vi "Teleop.vi"(10 "Match Info":T1={"Autonomous Elapsed Seconds"=0.0, "TeleOp Elapsed Seconds"=0.0, "Disabled Elapsed Seconds"=0.0, "Visited Autonomous"=FALSE, "Visited TeleOp"=FALSE, "Visited Disabled"=FALSE, "Autonomous Settings"={"Autonomous Style"=enum."Independent", "VI Refnum"=refnum}}, 11 "Call Context":T2) -> ()   [LabVIEW 2019]
doc: "This VI is called for each TeleOp packet received from the DS where the robot is not disabled. It is often used to read from the joysticks and update I/O or to update setpoints for timed control loops. It should complete and return within 20 milliseconds or it may miss DS packets."
uses:
  <vilib>/Rock Robotics/WPI/DriverStation/WPI_DriverStationDerivedRobotMode.ctl
  <vilib>/Rock Robotics/WPI/DriverStation/WPI_DriverStationMatch Info.ctl
  <vilib>/Rock Robotics/WPI/Utilities/WPI_GetSetVariantRefNum.vi
  Robot Global Data.vi
  <vilib>/Rock Robotics/Network Tables/NT Write Variant.vi
  <vilib>/Rock Robotics/Network Tables/NT Write Number.vi
  <vilib>/Rock Robotics/Network Tables/NT Write String.vi
  <vilib>/Rock Robotics/Network Tables/NT Write Boolean.vi
  <vilib>/Rock Robotics/Network Tables/NT Write Numeric Array.vi
  <vilib>/Rock Robotics/Network Tables/NT Write Boolean Array.vi
panel:
  in  "Blue Cal":cluster{"R":dbl, "G":dbl, "B":dbl}={"R"=0.143, "G"=0.427, "B"=0.429} caption="Blue Calibration"
  in  "Green Cal":cluster{"R":dbl, "G":dbl, "B":dbl}={"R"=0.197, "G"=0.561, "B"=0.24} caption="Green Calibration"
  in  "Red Cal":cluster{"R":dbl, "G":dbl, "B":dbl}={"R"=0.561, "G"=0.323, "B"=0.114} caption="Red Calibration"
  in  "Yellow Cal":cluster{"R":dbl, "G":dbl, "B":dbl}={"R"=0.361, "G"=0.524, "B"=0.113} caption="Yellow Calibration"
  out "Matched Color Name":string
  out "Match Confidence":dbl
  out "Measured Color":cluster{"R":dbl, "G":dbl, "B":dbl}
  out "error out 2":errorcluster
  out "Proximity":u16(graph)
  out "Color":u32(colorbox)
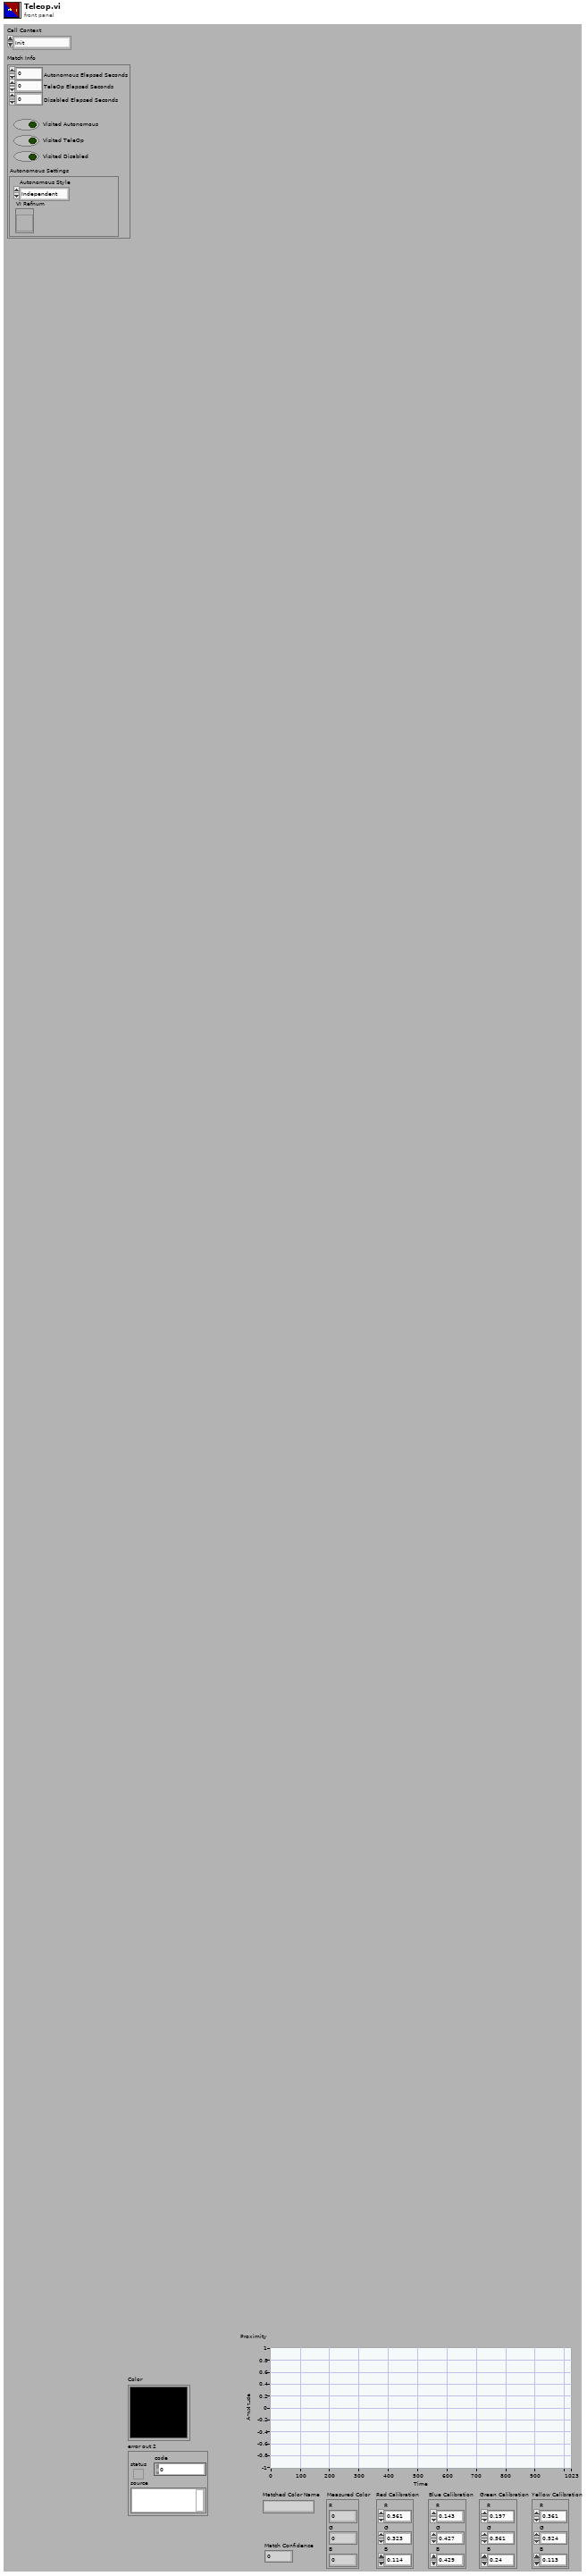
[diagram p1: front panel]
types:
  T1 = typedef "WPI_DriverStationMatch Info.ctl" = cluster{"Autonomous Elapsed Seconds":dbl, "TeleOp Elapsed Seconds":dbl, "Disabled Elapsed Seconds":dbl, "Visited Autonomous":bool, "Visited TeleOp":bool, "Visited Disabled":bool, "Autonomous Settings":cluster{"Autonomous Style":enum16{"Iterative", "Independent"}, "VI Refnum":refnum<vi>}}
  T2 = typedef "WPI_DriverStationDerivedRobotMode.ctl" = enum16{"Init", "Execute", "Stop"}
  T3 = typedef "WPI_JoystickDevRef.ctl" = cluster{"Device":T4}
  T4 = typedef "WPI_JoystickDeviceEnum.ctl" = enum16{"USB 0", "USB 1", "USB 2", "USB 3", "USB 4", "USB 5"}
  T5 = typedef "WPI_RobotDriveDevRef.ctl" = cluster{"DevStatus":errorcluster, "Motors[]":T6[], "Square Inputs":bool, "Max Output":dbl}
  T6 = typedef "WPI_MotorControlDeviceRef.ctl" = cluster{"DeviceStatus":errorcluster, "Type":T7, "PWM":cluster{"PWM Channel":T8, "DeadBand":T9}, "CAN":cluster{"Device Number":u8, "SetOutput VI Ref":variant, "GetOutput VI Ref":variant, "Enable VI Ref":variant, "Disable VI Ref":variant, "Data":variant}, "Invert":bool, "DIO PWM":cluster{"PWM \"Enable\" Channel":T8, "DIOChannel":T10, "PWM Rate":dbl}}
  T7 = typedef "WPI_MotorControlType.ctl" = enum16{"PWM", "CAN", "DIO PWM"}
  T8 = typedef "FPGA_DIOPWMChannel.ctl" = enum8{"PWM 0", "PWM 1", "PWM 2", "PWM 3", "PWM 4", "PWM 5", "PWM 6", "PWM 7", "PWM 8", "PWM 9", "PWM MXP 0", "PWM MXP 1", "PWM MXP 2", "PWM MXP 3", "PWM MXP 4", "PWM MXP 5", "PWM MXP 6", "PWM MXP 7", "PWM MXP 8", "PWM MXP 9", "Invalid"}
  T9 = typedef "WPI_PWMDeadband.ctl" = cluster{"Name":string, "maxPositivePwm":i32, "minPositivePwm":i32, "centerPwm":i32, "maxNegativePwm":i32, "minNegativePwm":i32, "angularRange":u16}
  T10 = typedef "FPGA_DIOChannel.ctl" = enum8{"DIO 0", "DIO 1", "DIO 2", "DIO 3", "DIO 4", "DIO 5", "DIO 6", "DIO 7", "DIO 8", "DIO 9", "DIO MXP 0", "DIO MXP 1", "DIO MXP 2", "DIO MXP 3", "DIO MXP 4", "DIO MXP 5", "DIO MXP 6", "DIO MXP 7", "DIO MXP 8", "DIO MXP 9", "DIO MXP 10", "DIO MXP 11", "DIO MXP 12", "DIO MXP 13", "DIO MXP 14", "DIO MXP 15", "SPI Port CS1", "SPI Port CS2", "SPI Port CS3", "SPI Port MISO", "SPI Port MOSI", "Invalid"}
  T11 = cluster{"JoystickDevRef":T3, "RobotDriveDevRef":T5}
  T12 = typedef "WPI_SwitchDevRef.ctl" = cluster{"DevStatus":errorcluster, "DIO Channel":T10, "CntIndex":T13, "Normally Closed":bool}
  T13 = typedef "FPGA_CounterCtrSystemIndex.ctl" = enum8{"Ctr 0", "Ctr 1", "Ctr 2", "Ctr 3", "Ctr 4", "Ctr 5", "Ctr 6", "Ctr 7", "Invalid"}
  T14 = typedef "Color Sensor V3 DevRef.ctl" = cluster{"I2CDevRef":T15}
  T15 = typedef "WPI_I2CDevRef.ctl" = cluster{"DevStatus":errorcluster, "Device Address":u8, "Handle":i32, "I2C Bus":T16}
  T16 = typedef "i2c_bus.ctl" = enum16{"I2C On-Board", "I2C MXP", "Invalid"}
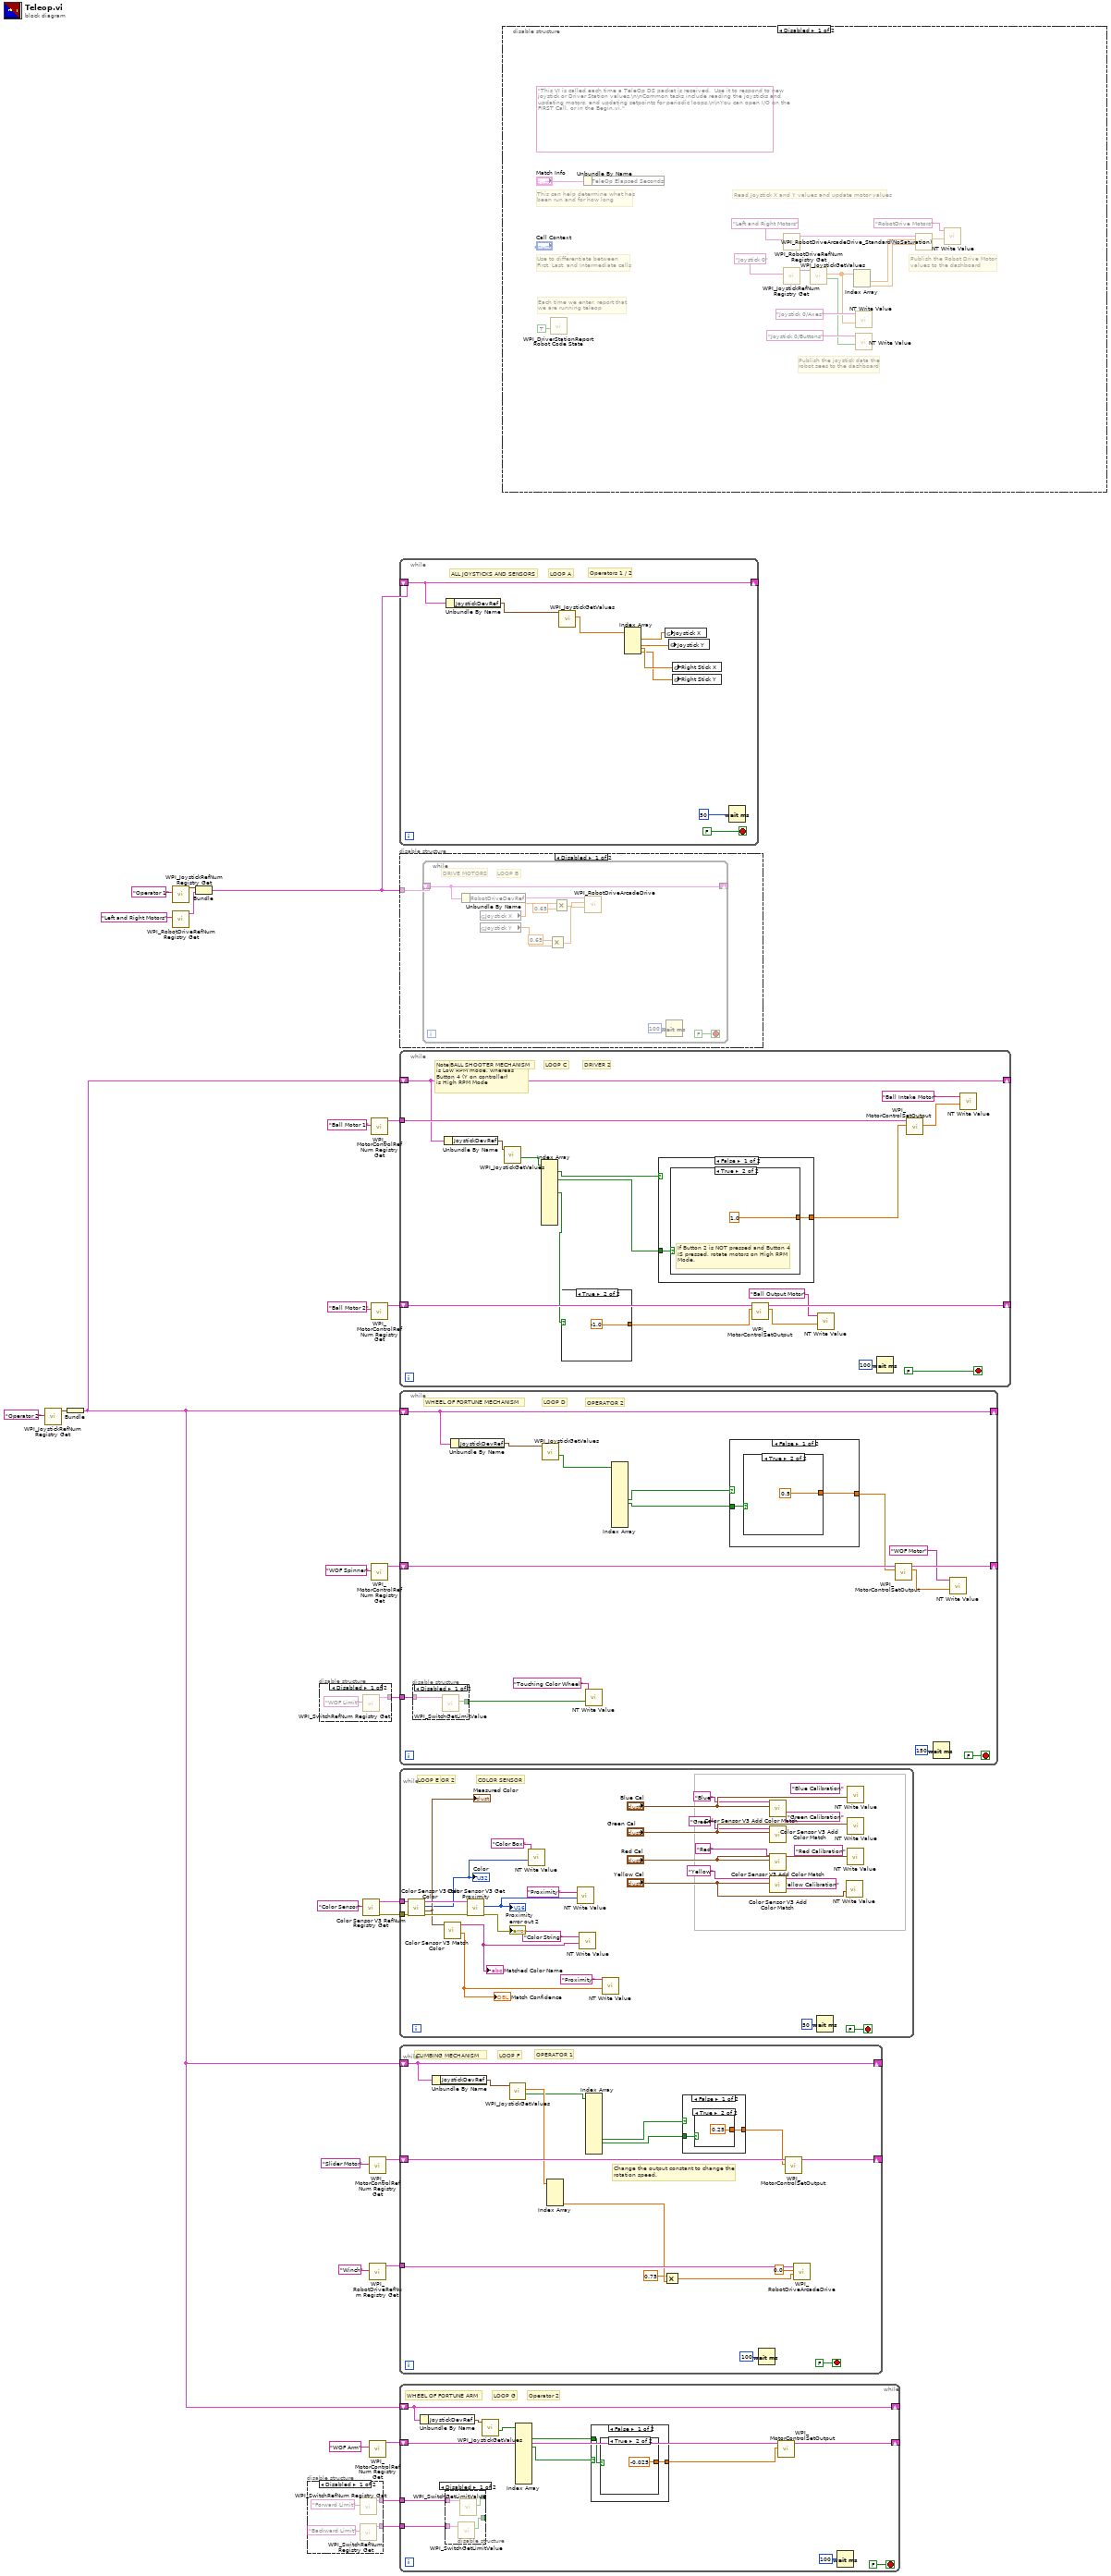
[diagram p0: block diagram]
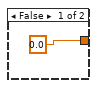
[diagram p4: hidden frame]
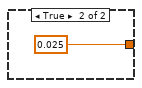
[diagram p5: hidden frame]
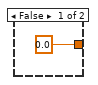
[diagram p7: hidden frame]
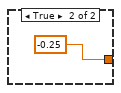
[diagram p8: hidden frame]
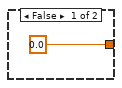
[diagram p12: hidden frame]
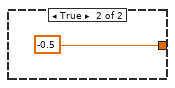
[diagram p13: hidden frame]
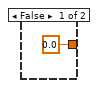
[diagram p14: hidden frame]
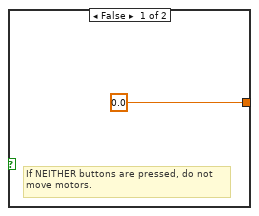
[diagram p15: hidden frame]
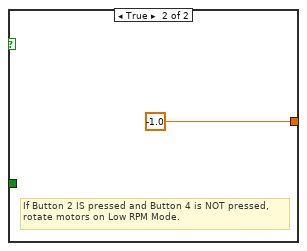
[diagram p16: hidden frame]
diagram:
  n1 = call <vilib>:"WPI_JoystickRefNum Registry Get.vi"("refnum name"="Operator 2") -> ("JoystickDevRef"=w5:T3)  [unwired: 9 in, 1 out]
  n2 = Bundle("JoystickDevRef"=w5) -> (w1:cluster{"JoystickDevRef":T3})  [unwired: 1 in]
  n3 = call <vilib>:"WPI_JoystickRefNum Registry Get.vi"("refnum name"="Operator 1") -> ("JoystickDevRef"=w24:T3)  [unwired: 1 in, 9 out]
  n4 = call <vilib>:"WPI_RobotDriveRefNum Registry Get.vi"("refnum name"="Left and Right Motors") -> ("RobotDriveDevRef"=w23:T5)  [unwired: 1 in, 9 out]
  n5 = Bundle("JoystickDevRef"=w24, "RobotDriveDevRef"=w23) -> (w2:T11)  [unwired: 1 out]
  n6 = disable-structure shown="Disabled" {
    disable-tunnel: [w28 _] -> w8
    disable-tunnel: [w27 _] -> w7
    frame Disabled {
      n7 = call <vilib>:"WPI_SwitchRefNum Registry Get.vi"("refnum name"="Forward Limit") -> ("SwitchDevRef"=w28:T12)  [unwired: 9 in, 1 out]
      n8 = call <vilib>:"WPI_SwitchRefNum Registry Get.vi"("refnum name"="Backward Limit") -> ("SwitchDevRef"=w27:T12)  [unwired: 9 in, 1 out]
    }
    frame Enabled {
    }
  }
  n9 = disable-structure shown="Disabled" {
    disable-tunnel: [w31 _] -> w13
    frame Disabled {
      n10 = call <vilib>:"WPI_SwitchRefNum Registry Get.vi"("refnum name"="WOF Limit") -> ("SwitchDevRef"=w31:T12)  [unwired: 9 in, 1 out]
    }
    frame Enabled {
    }
  }
  n11 = call <vilib>:"Color Sensor V3 RefNum Registry Get.vi"("refnum name"="Color Sensor") -> ("error out"=w17:errorcluster, "ColorSensorDevRef"=w18:T14)  [unwired: 9 in]
  n12 = call <vilib>:"WPI_MotorControlRefNum Registry Get.vi"("refnum name"="Slider Motor") -> ("MotorControlDevRef"=w12:T6)  [unwired: 9 in, 1 out]
  n13 = call <vilib>:"WPI_RobotDriveRefNum Registry Get.vi"("refnum name"="Winch") -> ("RobotDriveDevRef"=w4:T5)  [unwired: 9 in, 1 out]
  n14 = call <vilib>:"WPI_MotorControlRefNum Registry Get.vi"("refnum name"="WOF Arm") -> ("MotorControlDevRef"=w10:T6)  [unwired: 9 in, 1 out]
  n15 = call <vilib>:"WPI_MotorControlRefNum Registry Get.vi"("refnum name"="Ball Motor 1") -> ("MotorControlDevRef"=w21:T6)  [unwired: 9 in, 1 out]
  n16 = call <vilib>:"WPI_MotorControlRefNum Registry Get.vi"("refnum name"="Ball Motor 2") -> ("MotorControlDevRef"=w14:T6)  [unwired: 9 in, 1 out]
  n17 = call <vilib>:"WPI_MotorControlRefNum Registry Get.vi"("refnum name"="WOF Spinner") -> ("MotorControlDevRef"=w19:T6)  [unwired: 9 in, 1 out]
  n18 = while {
    shift-right: [w40] -> _
    shift-left: w2 -> [w40]
    stop <- FALSE stop-if-true
    # "Operators 1 / 2"
    # "LOOP A"
    # "ALL JOYSTICKS AND SENSORS"
    n19 = Unbundle By Name(w40) -> ("JoystickDevRef"=w39:T3)
    n20 = call <vilib>:"WPI_JoystickGetValues.vi"("JoystickDevRef"=w39) -> ("Axes"=w38:dbl[])  [unwired: 6 in, 4 out]
    n21 = Index Array(array=w38) -> (element #1=w36:dbl, element #2=w37:dbl, element #3=w34:dbl, element #4=w33:dbl)  [unwired: 4 in]
    n22 = global write "Robot Global Data.vi" "Joystick X"(w36) -> ()
    n23 = global write "Robot Global Data.vi" "Joystick Y"(w37) -> ()
    n24 = global write "Robot Global Data.vi" "Right Stick X"(w34) -> ()
    n25 = global write "Robot Global Data.vi" "Right Stick Y"(w33) -> ()
    n26 = Wait (ms)(milliseconds to wait=u32 50) -> ()  [unwired: 1 out]
  }
  n27 = disable-structure shown="Disabled" {
    disable-tunnel: w2 -> [w42 _]
    frame Disabled {
      n28 = while {
        shift-right: [w50] -> _
        shift-left: w42 -> [w50]
        stop <- FALSE stop-if-true
        # "DRIVE MOTORS"
        # "LOOP B"
        n29 = Unbundle By Name(w50) -> ("RobotDriveDevRef"=w49:T5)
        n30 = global read "Robot Global Data.vi" "Joystick X"() -> (w47:dbl)
        n31 = global read "Robot Global Data.vi" "Joystick Y"() -> (w48:dbl)
        n32 = Multiply(x=0.65, y=w48) -> (x*y=w44:dbl)
        n33 = Multiply(x=w47, y=0.65) -> (x*y=w43:dbl)
        n34 = call-poly <vilib>:"WPI_RobotDriveArcadeDrive.vi"("Y axis value"=w44, "X axis value"=w43, "RobotDriveDevRef"=w49) -> ()  [unwired: 6 in, 3 out]
        n35 = Wait (ms)(milliseconds to wait=u32 100) -> ()  [unwired: 1 out]
      }
    }
    frame Enabled {
    }
  }
  n36 = while {
    tunnel: w21 -> [w67]
    shift-right: [w63] -> _
    shift-left: w14 -> [w64]
    shift-right: [w54] -> _
    shift-left: w1 -> [w54]
    stop <- FALSE stop-if-true
    # "DRIVER 2"
    # "LOOP C"
    # "Note: Button 2 (A on controller) \nis Low RPM mode, whereas \nButton 4 (Y on controller)\nis High RPM Mode"
    # "BALL SHOOTER MECHANISM"
    n37 = Unbundle By Name(w54) -> ("JoystickDevRef"=w53:T3)
    n38 = call <vilib>:"WPI_JoystickGetValues.vi"("JoystickDevRef"=w53) -> ("Buttons"=w65:bool[])  [unwired: 6 in, 4 out]
    n39 = Index Array(array=w65) -> (element #1=w62:bool, element #3=w61:bool, element #6=w59:bool)  [unwired: 13 in, 10 out]
    n40 = case shown="True" w59 {
      tunnel: [0.0 ("Output") -1.0 ("Output")] -> w60
      frame False {
      }
      frame True {
      }
    }
    n41 = case shown="False" w62 {
      tunnel: [w73 -1.0 ("Output")] -> w66
      tunnel: w61 -> [w72 _]
      frame False {
        n42 = case shown="True" w72 {
          tunnel: [0.0 ("Output") 1.0 ("Output")] -> w73
          frame False {
            # "If NEITHER buttons are pressed, do not\nmove motors."
          }
          frame True {
            # "If Button 2 is NOT pressed and Button 4\nIS pressed, rotate motors on High RPM\nMode."
          }
        }
      }
      frame True {
        # "If Button 2 IS pressed and Button 4 is NOT pressed,\nrotate motors on Low RPM Mode."
      }
    }
    n43 = call <vilib>:"WPI_MotorControlSetOutput.vi"("Output"=w60, "MotorControlDevRef"=w64) -> ("Motor Output"=w56:dbl, "MotorControlDevRef"=w63:T6)  [unwired: 7 in, 1 out]
    n44 = call-poly <vilib>:"NT Write Value.vi"("Numeric"=w56, "Name"="Ball Output Motor") -> ()  [unwired: 9 in, 1 out]
    n45 = Wait (ms)(milliseconds to wait=u32 100) -> ()  [unwired: 1 out]
    n46 = call <vilib>:"WPI_MotorControlSetOutput.vi"("Output"=w66, "MotorControlDevRef"=w67) -> ("Motor Output"=w58:dbl)  [unwired: 7 in, 2 out]
    n47 = call-poly <vilib>:"NT Write Value.vi"("Numeric"=w58, "Name"="Ball Intake Motor") -> ()  [unwired: 9 in, 1 out]
  }
  n48 = while {
    shift-right: [w89] -> _
    shift-left: w19 -> [w90]
    tunnel: w13 -> [w86]
    shift-right: [w78] -> _
    shift-left: w1 -> [w78]
    stop <- FALSE stop-if-true
    # "OPERATOR 2"
    # "LOOP D"
    # "WHEEL OF FORTUNE MECHANISM"
    n49 = disable-structure shown="Disabled" {
      disable-tunnel: w86 -> [w93 _]
      disable-tunnel: [w92 _] -> w84
      frame Disabled {
        n50 = call <vilib>:"WPI_SwitchGetLimitValue.vi"("SwitchDevRef"=w93) -> ("Switch Pressed"=w92:bool)  [unwired: 8 in, 2 out]
      }
      frame Enabled {
      }
    }
    n51 = Unbundle By Name(w78) -> ("JoystickDevRef"=w77:T3)
    n52 = call <vilib>:"WPI_JoystickGetValues.vi"("JoystickDevRef"=w77) -> ("Buttons"=w83:bool[])  [unwired: 6 in, 4 out]
    n53 = call-poly <vilib>:"NT Write Value.vi"("Boolean"=w84, "Name"="Touching Color Wheel") -> ()  [unwired: 9 in, 1 out]
    n54 = Index Array(array=w83) -> (element #7=w82:bool, element #8=w81:bool)  [unwired: 13 in, 11 out]
    n55 = case shown="False" w82 {
      tunnel: [w95 -0.5 ("Output")] -> w88
      tunnel: w81 -> [w94 _]
      frame False {
        n56 = case shown="True" w94 {
          tunnel: [0.0 ("Output") 0.5 ("Output")] -> w95
          frame False {
          }
          frame True {
          }
        }
      }
      frame True {
      }
    }
    n57 = call <vilib>:"WPI_MotorControlSetOutput.vi"("Output"=w88, "MotorControlDevRef"=w90) -> ("Motor Output"=w80:dbl, "MotorControlDevRef"=w89:T6)  [unwired: 7 in, 1 out]
    n58 = Wait (ms)(milliseconds to wait=u32 150) -> ()  [unwired: 1 out]
    n59 = call-poly <vilib>:"NT Write Value.vi"("Numeric"=w80, "Name"="WOF Motor") -> ()  [unwired: 9 in, 1 out]
  }
  n60 = while {
    tunnel: w18 -> [w108]
    tunnel: w17 -> [w107]
    stop <- FALSE stop-if-true
    (unwired) "Yellow Calibration" ("Name")
    (unwired) "Red Calibration" ("Name")
    (unwired) "Green Calibration" ("Name")
    (unwired) "Blue Calibration" ("Name")
    # "OPERATOR 2"
    # "LOOP E"
    # "COLOR SENSOR"
    n61 = call <vilib>:"Color Sensor V3 Get Color.vi"("error in (no error)"=w107, "ColorSensorDevRef"=w108) -> ("error out"=w122:errorcluster, "Normalized Color"=w119:cluster{"R":dbl, "G":dbl, "B":dbl}, "Color"=w116:u32, "ColorSensorDevRef out"=w121:T14)  [unwired: 6 in]
    "Color" <- w116
    "Measured Color" <- w119
    n62 = call <vilib>:"Color Sensor V3 Match Color.vi"("Measured Color"=w119) -> ("Confidence"=w112:dbl, "Matched Color Name"=w110:string)  [unwired: 8 in, 1 out]
    "Match Confidence" <- w112
    "Matched Color Name" <- w110
    n63 = call <vilib>:"Color Sensor V3 Get Proximity.vi"("error in (no error)"=w122, "ColorSensorDevRef"=w121) -> ("error out"=→"error out 2":errorcluster, "Proximity"=w114:u16)  [unwired: 7 in, 1 out]
    "Proximity" <- w114
    n64 = call-poly <vilib>:"NT Write Value.vi"("Numeric"=w116, "Name"="Color Box") -> ()  [unwired: 9 in, 1 out]
    n65 = call-poly <vilib>:"NT Write Value.vi"("Numeric"=w114, "Name"="Proximity") -> ()  [unwired: 9 in, 1 out]
    n66 = call-poly <vilib>:"NT Write Value.vi"("String"=w110, "Name"="Color String") -> ()  [unwired: 9 in, 1 out]
    n67 = call-poly <vilib>:"NT Write Value.vi"("Numeric"=w112, "Name"="Proximity") -> ()  [unwired: 9 in, 1 out]
    n68 = call <vilib>:"Color Sensor V3 Add Color Match.vi"("Color"="Blue Cal", "Name"="Blue") -> ()  [unwired: 10 in]
    n69 = call <vilib>:"Color Sensor V3 Add Color Match.vi"("Color"="Green Cal", "Name"="Green") -> ()  [unwired: 10 in]
    n70 = call <vilib>:"Color Sensor V3 Add Color Match.vi"("Color"="Red Cal", "Name"="Red") -> ()  [unwired: 10 in]
    n71 = call <vilib>:"Color Sensor V3 Add Color Match.vi"("Color"="Yellow Cal", "Name"="Yellow") -> ()  [unwired: 10 in]
    n72 = Wait (ms)(milliseconds to wait=u32 50) -> ()  [unwired: 1 out]
    n73 = call-poly <vilib>:"NT Write Value.vi"("Variant"="Yellow Cal") -> ()  [unwired: 10 in, 1 out]
    n74 = call-poly <vilib>:"NT Write Value.vi"("Variant"="Red Cal") -> ()  [unwired: 10 in, 1 out]
    n75 = call-poly <vilib>:"NT Write Value.vi"("Variant"="Blue Cal") -> ()  [unwired: 10 in, 1 out]
    n76 = call-poly <vilib>:"NT Write Value.vi"("Variant"="Green Cal") -> ()  [unwired: 10 in, 1 out]
  }
  n77 = while {
    shift-right: [w123] -> _
    shift-left: w12 -> [w138]
    tunnel: w4 -> [w133]
    shift-right: [w125] -> _
    shift-left: w1 -> [w125]
    stop <- FALSE stop-if-true
    # "Change the output constant to change the\nrotation speed."
    # "OPERATOR 1"
    # "LOOP F"
    # "CLIMBING MECHANISM"
    n78 = Unbundle By Name(w125) -> ("JoystickDevRef"=w124:T3)
    n79 = call <vilib>:"WPI_JoystickGetValues.vi"("JoystickDevRef"=w124) -> ("Buttons"=w128:bool[], "Axes"=w134:dbl[])  [unwired: 6 in, 3 out]
    n80 = Index Array(array=w134) -> (element #4=w130:dbl)  [unwired: 4 in, 3 out]
    n81 = Index Array(array=w128) -> (element #9=w127:bool, element #10=w126:bool)  [unwired: 12 in, 10 out]
    n82 = Multiply(x=0.75, y=w130) -> (x*y=w131:dbl)
    n83 = case shown="False" w127 {
      tunnel: [w140 -0.25 ("Output")] -> w136
      tunnel: w126 -> [w139 _]
      frame False {
        n84 = case shown="True" w139 {
          tunnel: [0.0 ("Output") 0.25 ("Output")] -> w140
          frame False {
          }
          frame True {
          }
        }
      }
      frame True {
      }
    }
    n85 = Wait (ms)(milliseconds to wait=u32 100) -> ()  [unwired: 1 out]
    n86 = call <vilib>:"WPI_MotorControlSetOutput.vi"("Output"=w136, "MotorControlDevRef"=w138) -> ("MotorControlDevRef"=w123:T6)  [unwired: 7 in, 2 out]
    n87 = call-poly <vilib>:"WPI_RobotDriveArcadeDrive.vi"("Y axis value"=w131, "X axis value"=0.0, "RobotDriveDevRef"=w133) -> ()  [unwired: 6 in, 3 out]
  }
  n88 = while {
    shift-right: [w154] -> _
    shift-left: w10 -> [w153]
    tunnel: w8 -> [w151]
    tunnel: w7 -> [w150]
    shift-right: [w145] -> _
    shift-left: w1 -> [w145]
    stop <- FALSE stop-if-true
    # "LOOP G"
    # "Operator 2"
    # "WHEEL OF FORTUNE ARM"
    n89 = Unbundle By Name(w145) -> ("JoystickDevRef"=w144:T3)
    n90 = disable-structure shown="Disabled" {
      disable-tunnel: w151 -> [w164 _]
      disable-tunnel: w150 -> [w163 _]
      disable-tunnel: [w162 _] -> _
      disable-tunnel: [w161 _] -> _
      frame Disabled {
        n91 = call <vilib>:"WPI_SwitchGetLimitValue.vi"("SwitchDevRef"=w163) -> ("Switch Pressed"=w161:bool)  [unwired: 8 in, 2 out]
        n92 = call <vilib>:"WPI_SwitchGetLimitValue.vi"("SwitchDevRef"=w164) -> ("Switch Pressed"=w162:bool)  [unwired: 8 in, 2 out]
      }
      frame Enabled {
      }
    }
    n93 = call <vilib>:"WPI_JoystickGetValues.vi"("JoystickDevRef"=w144) -> ("Buttons"=w152:bool[])  [unwired: 6 in, 4 out]
    n94 = Index Array(array=w152) -> (element #2=w147:bool, element #4=w149:bool)  [unwired: 12 in, 10 out]
    n95 = case shown="False" w149 {
      tunnel: [w156 0.025 ("Output")] -> w148
      tunnel: w147 -> [w157 _]
      frame False {
        n96 = case shown="True" w157 {
          tunnel: [0.0 ("Output") -0.025 ("Output")] -> w156
          frame False {
          }
          frame True {
          }
        }
      }
      frame True {
      }
    }
    n97 = call <vilib>:"WPI_MotorControlSetOutput.vi"("Output"=w148, "MotorControlDevRef"=w153) -> ("MotorControlDevRef"=w154:T6)  [unwired: 7 in, 2 out]
    n98 = Wait (ms)(milliseconds to wait=u32 100) -> ()  [unwired: 1 out]
  }
  n99 = disable-structure shown="Disabled" {
    frame Disabled {
      (unwired) "This VI is called each time a TeleOp DS packet is received.  Use it to respond to new joystick or Driver Station values.\n\nCommon tasks include reading the joysticks and updating motors, and updating setpoints for periodic loops.\n\nYou can open I/O on the FIRST Call, or in the Begin.vi."
      # "Publish the Robot Drive Motor\nvalues to the dashboard"
      # "Publish the joystick data the\nrobot sees to the dashboard"
      # "Each time we enter, report that\nwe are running teleop"
      # "Use to differentiate between\nFirst, Last, and Intermediate calls"
      # "This can help determine what has\nbeen run and for how long"
      # "Read Joystick X and Y values and update motor values"
      n100 = call <vilib>:"WPI_DriverStationReport Robot Code State.vi"("TeleOp"=TRUE ("Autonomous")) -> ()  [unwired: 10 in, 1 out]
      n101 = Unbundle By Name("Match Info") -> ()  [unwired: 1 out]
      n102 = call <vilib>:"WPI_RobotDriveRefNum Registry Get.vi"("refnum name"="Left and Right Motors") -> ("RobotDriveDevRef"=w176:T5)  [unwired: 1 in, 9 out]
      n103 = call <vilib>:"WPI_JoystickRefNum Registry Get.vi"("refnum name"="Joystick 0") -> ("JoystickDevRef"=w173:T3)  [unwired: 1 in, 9 out]
      n104 = call <vilib>:"WPI_JoystickGetValues.vi"("JoystickDevRef"=w173) -> ("Buttons"=w167:bool[], "Axes"=w168:dbl[])  [unwired: 6 in, 3 out]
      n105 = Index Array(array=w168) -> (element #1=w175:dbl, element #2=w171:dbl)  [unwired: 2 in]
      n106 = call-poly <vilib>:"NT Write Value.vi"("Numeric Array"=w168, "Name"="Joystick 0/Axes") -> ()  [unwired: 9 in, 1 out]
      n107 = call-poly <vilib>:"NT Write Value.vi"("Boolean Array"=w167, "Name"="Joystick 0/Buttons") -> ()  [unwired: 9 in, 1 out]
      n108 = call <vilib>:"WPI_RobotDriveArcadeDrive_Standard(NoSaturation).vi"("Y axis value"=w171, "X axis value"=w175, "RobotDriveDevRef"=w176) -> ("Motor Values"=w166:dbl[])  [unwired: 1 in, 7 out]
      n109 = call-poly <vilib>:"NT Write Value.vi"("Numeric Array"=w166, "Name"="RobotDrive Motors") -> ()  [unwired: 9 in, 1 out]
    }
    frame Enabled {
    }
  }
